vi "GetValue(Channel).vi"(11 "Cluster":T1) -> ()   [LabVIEW 2025, in "DAQ_Module.lvlib" / "DAQ_Module.lvclass"]
uses:
  DAQ_Module.lvclass
  DAQ_Module.lvclass/DAQ_Module.ctl
  c6eacb99-7883-44c6-93b4-a96c8fa4f5d2.vi
  12374cb4-71a1-49e9-9cec-671213deaeb6.vi
  fa96c98e-2ad4-4b53-a526-4274ed38981d.vi
  DAQ_Task_Type.ctl
  DAQ_SampleRateConfig.ctl
  DAQ_HW_Type.ctl
  DAQ_Task_Config.ctl
  DAQ_Config.ctl
  DAQ_AI_Task_Config.ctl
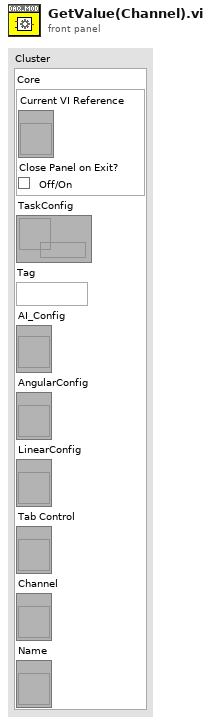
[diagram p1: front panel]
types:
  T1 = cluster{"Core":cluster{"Current VI Reference":refnum<vi>, "Close Panel on Exit?":bool}, "TaskConfig":refnum<data-value>, "Tag":string, "AI_Config":refnum<vi>, "AngularConfig":refnum<vi>, "LinearConfig":refnum<vi>, "Tab Control":refnum<vi>, "Channel":refnum<vi>, "Name":refnum<vi>}
  T2 = typedef "DAQ_Module.lvlib/DAQ_Module.lvclass/DAQ_Config.ctl" = map{string, T3}
  T3 = typedef "DAQ_Module.lvlib/DAQ_Module.lvclass/DAQ_Task_Config.ctl" = cluster{"Drive":T4, "TaskType":T5, "PhysicalChannels":string, "SampleRateConfiguration":T6, "ChannelConfig":map{string, cluster{"Name":string, "Config":string}}, "Enable":bool, "ShowPanel":bool}
  T4 = typedef "DAQ_Module.lvlib/DAQ_Module.lvclass/DAQ_HW_Type.ctl" = enum16{"NI_DAQmx", "Simulated_DAQ"}
  T5 = typedef "DAQ_Module.lvlib/DAQ_Module.lvclass/DAQ_Task_Type.ctl" = enum16{"AI", "Linear", "Angular", "AO"}
  T6 = typedef "DAQ_Module.lvlib/DAQ_Module.lvclass/DAQ_SampleRateConfig.ctl" = cluster{"SampleRate":dbl, "SamplesPerChannel":u32, "SamplesPerRead":i32, "SampleMode":i32, "Clock Source":string}
  T7 = map{string, cluster{"Name":string, "Config":string}}
  T8 = typedef "DAQ_Module.lvlib/DAQ_Module.lvclass/DAQ_Linear_Task_Config.ctl" = cluster{"decoding type":i32, "units":i32, "distance per pulse":dbl, "initial position":dbl, "z index enable":bool, "z index value":dbl, "z index phase":i32, "CI_Encoder_A_InputTerm":string, "CI_Encoder_B_InputTerm":string, "CI_Encoder_Z_InputTerm":string}
  T9 = typedef "DAQ_Module.lvlib/DAQ_Module.lvclass/DAQ_Angular_Task_Config.ctl" = cluster{"decoding type":i32, "units":i32, "pulses per revolution":u32, "initial angle":dbl, "z index enable":bool, "z index value":dbl, "z index phase":i32, "CI_Encoder_A_InputTerm":string, "CI_Encoder_B_InputTerm":string, "CI_Encoder_Z_InputTerm":string}
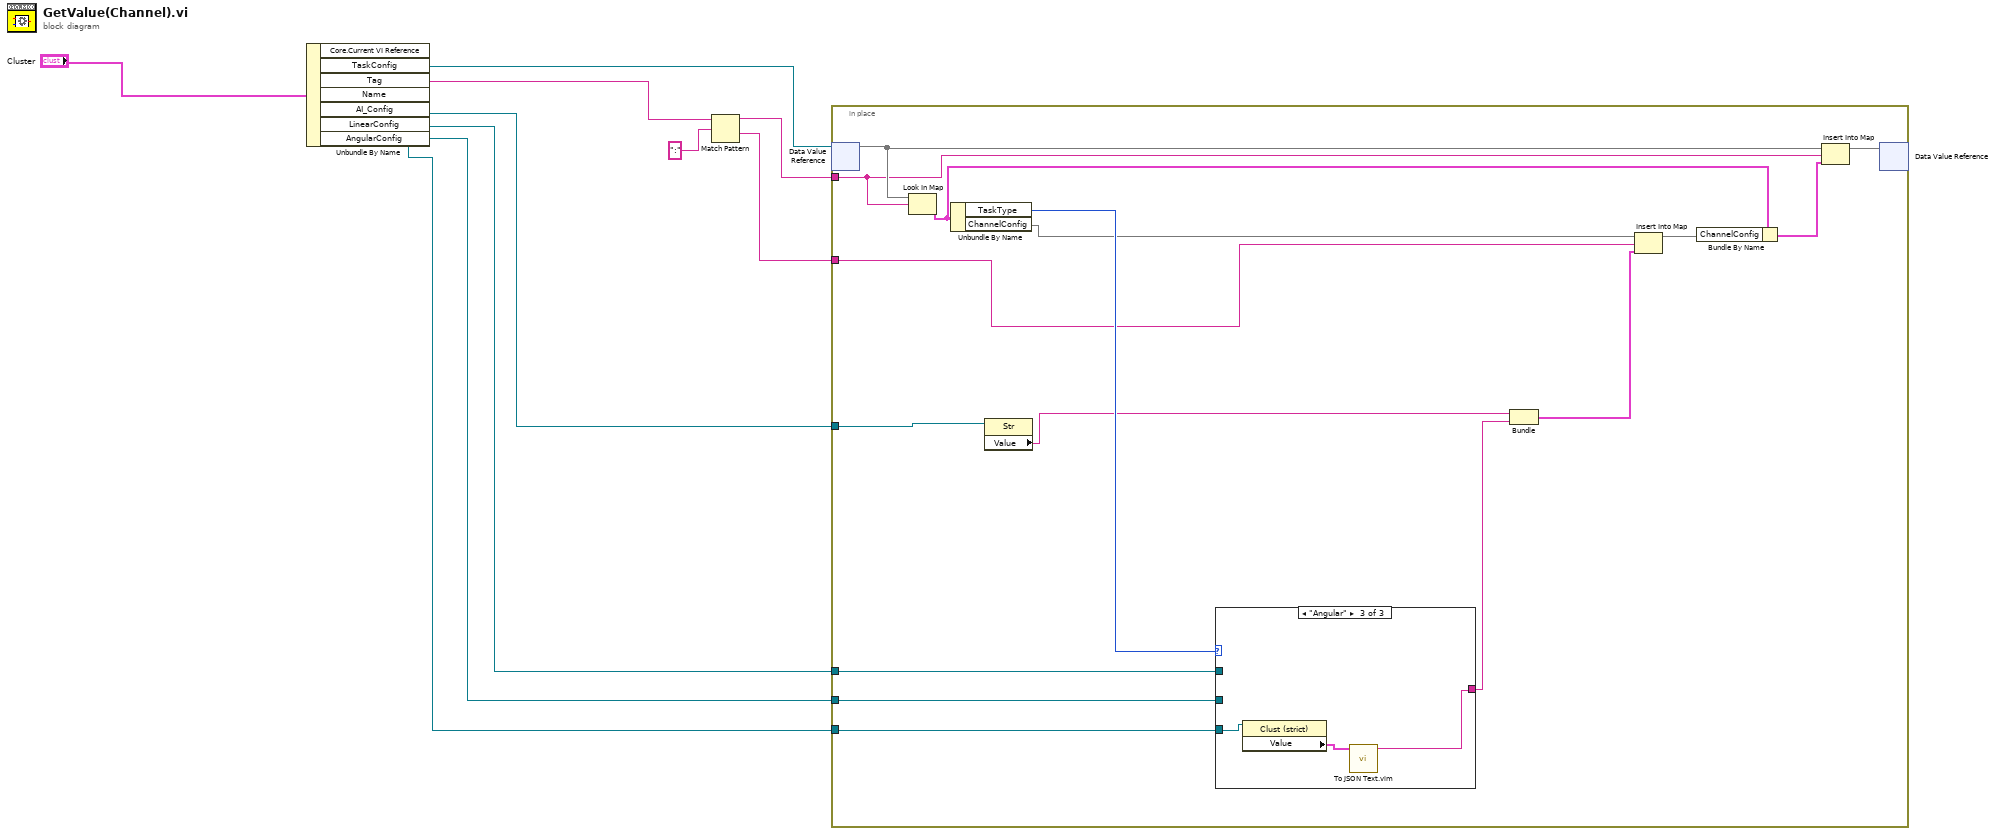
[diagram p0: block diagram]
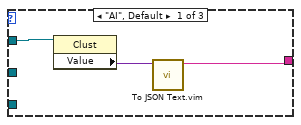
[diagram p2: hidden frame]
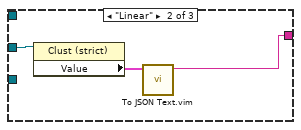
[diagram p3: hidden frame]
diagram:
  n1 = Unbundle By Name("Cluster") -> ("TaskConfig"=w7:refnum<data-value>, "Tag"=w6:string, "Name"=w5:refnum<vi>, "AI_Config"=w4:refnum<vi>, "LinearConfig"=w3:refnum<vi>, "AngularConfig"=w2:refnum<vi>)  [unwired: 1 out]
  n2 = Match Pattern(string=w6, regular expression=":") -> (before substring=w9:string, after substring=w8:string)  [unwired: 1 in, 2 out]
  n3 = in-place {
    in-place-border: w9 -> [w15]
    in-place-border: w8 -> [w20]
    in-place-border: w5 -> [w26]
    in-place-border: w4 -> [w24]
    in-place-border: w3 -> [w23]
    in-place-border: w2 -> [w22]
    n4 = in-place-dvr #1(w7) -> (w16:T2)  [unwired: 1 out]
    n5 = Look In Map(map=w16, key=w15) -> (value=w14:T3)  [unwired: 1 in, 1 out]
    n6 = Unbundle By Name(w14) -> ("TaskType"=w25:T5, "ChannelConfig"=w21:T7)
    n7 = property class="Str"(reference=w26) -> ("Value"=w19:string)  [unwired: 1 in, 2 out]
    n8 = case shown="\"Angular\"" w25 {
      tunnel: w24 -> [w29 _ _]
      tunnel: w23 -> [_ w32 _]
      tunnel: w22 -> [_ _ w35]
      tunnel: [w27 w30 w33] -> w18
      frame "AI", Default {
        n9 = property class="Clust"(reference=w29) -> ("Value"=w28:variant)  [unwired: 1 in, 2 out]
        n10 = call "To JSON Text.vim"("Anything"=w28) -> ("<JSON>"=w27:string)  [unwired: 9 in, 1 out]
      }
      frame "Linear" {
        n11 = property class="Clust (strict)"(reference=w32) -> ("Value"=w31:T8)  [unwired: 1 in, 2 out]
        n12 = call "To JSON Text.vim"("Anything"=w31) -> ("<JSON>"=w30:string)  [unwired: 9 in, 1 out]
      }
      frame "Angular" {
        n13 = property class="Clust (strict)"(reference=w35) -> ("Value"=w34:T9)  [unwired: 1 in, 2 out]
        n14 = call "To JSON Text.vim"("Anything"=w34) -> ("<JSON>"=w33:string)  [unwired: 9 in, 1 out]
      }
    }
    n15 = Bundle("Value"=w19, "<JSON>"=w18) -> (w17:cluster{"Value":string, "<JSON>":string})  [unwired: 1 in]
    n16 = Insert Into Map(map in=w21, key=w20, value=w17) -> (map out=w13:T7)  [unwired: 2 out]
    n17 = Bundle By Name(cluster=w14, "ChannelConfig"=w13) -> (w12:T3)
    n18 = Insert Into Map(map in=w16, key=w15, value=w12) -> (map out=w11:T2)  [unwired: 2 out]
    n19 = in-place-dvr #1(w11) -> ()  [unwired: 2 out]
  }
